vi "selectROI.vi"() -> ()   [LabVIEW 2010]
uses:
  <vilib>/Utility/miscctls.llb/LVPoint32TypeDef.ctl
  <vilib>/measure/NI_MABase.lvlib
panel:
  out "bottom":i32
  out "right":i32
  out "top":i32
  out "Left":i32
  out "bottom":i16
  out "right":i16
  out "top":i16
  out "left":i16
  in  "signal type":T1(ring)
  in  "amplitude":dbl(slide)=10.0 scale=0.0..10.0
  in  "frequency":dbl(slide)=9.923664122137405 scale=0.0..100.0
  in  "stop":bool
  out "Waveform Graph":waveform(dbl)(graph)={"t0"=timestamp(22.0 s since 1904-01-01), "dt"=0.001, "Y"=array[1000 elements]}
  # "plot bounds"
  # "ROI bounds"
  # "Define the graph rectangle by selecting an area with mouse"
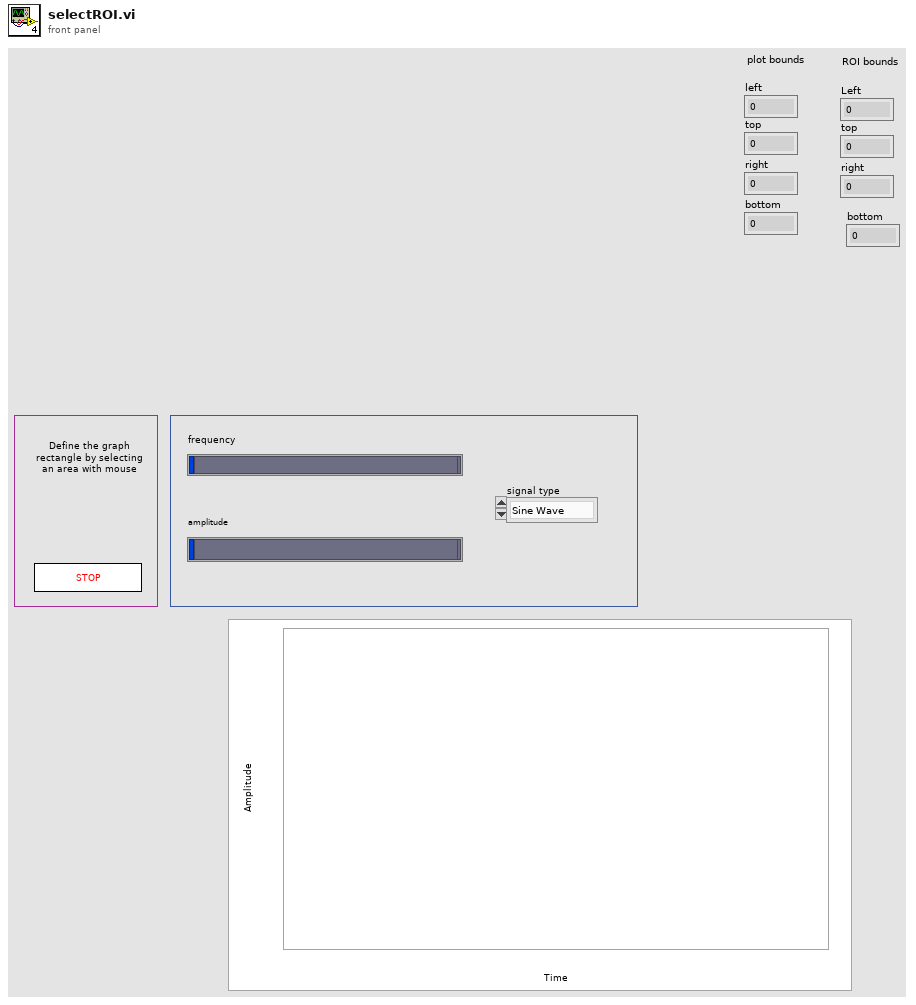
[diagram p1: front panel]
types:
  T1 = enum16{"Sine Wave", "Triangle Wave", "Square Wave", "Sawtooth Wave"}
  T2 = typedef "LVPoint32TypeDef.ctl" = cluster{"Horizontal":i32, "Vertical":i32}
  T3 = typedef "LVRectTypeDef.ctl" = cluster{"left":i16, "top":i16, "right":i16, "bottom":i16}
  T4 = cluster{"Width":i16, "Style":enum32{"Solid", "Dash", "Dot", "DashDot", "DashDotDot"}}
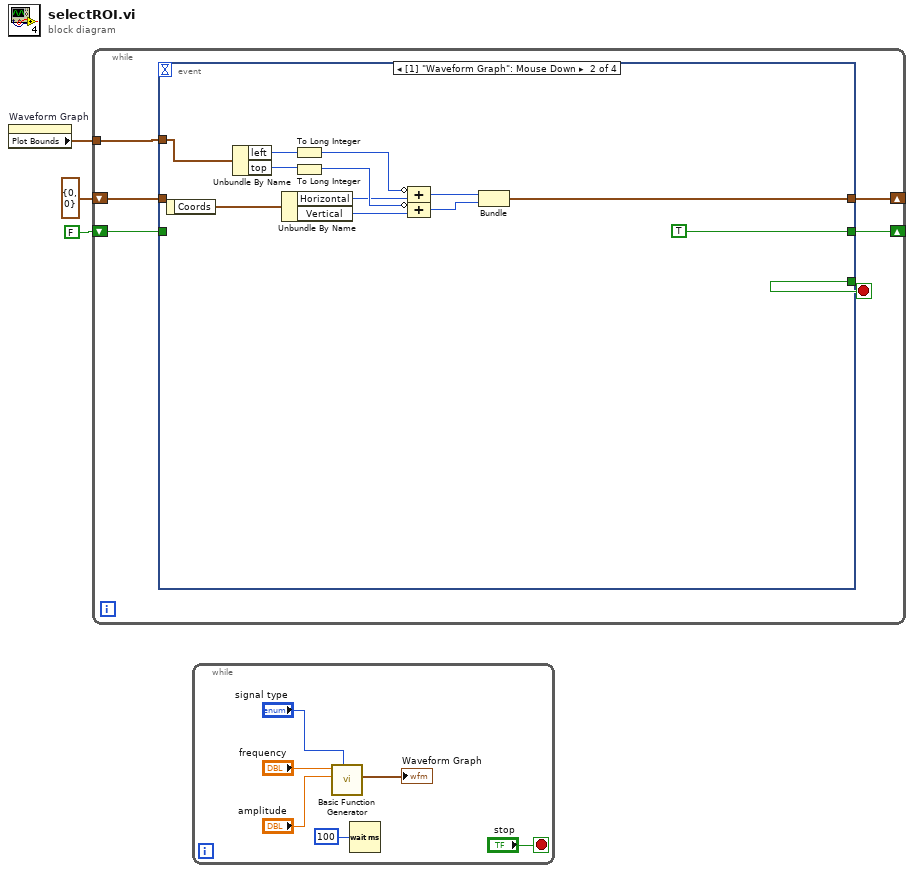
[diagram p0: block diagram]
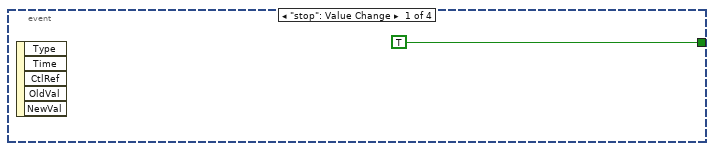
[diagram p2: hidden frame]
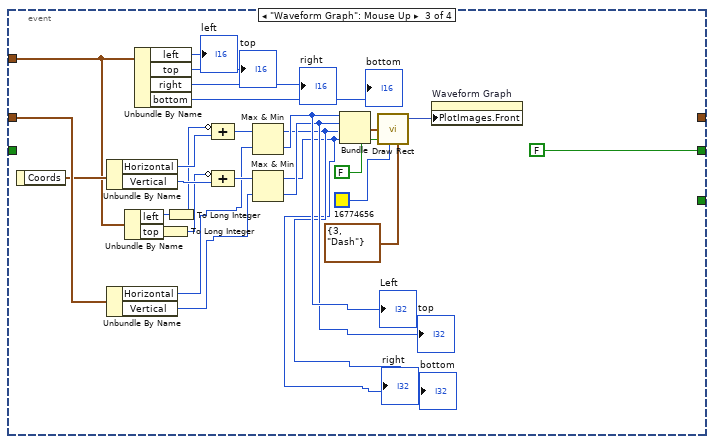
[diagram p3: hidden frame]
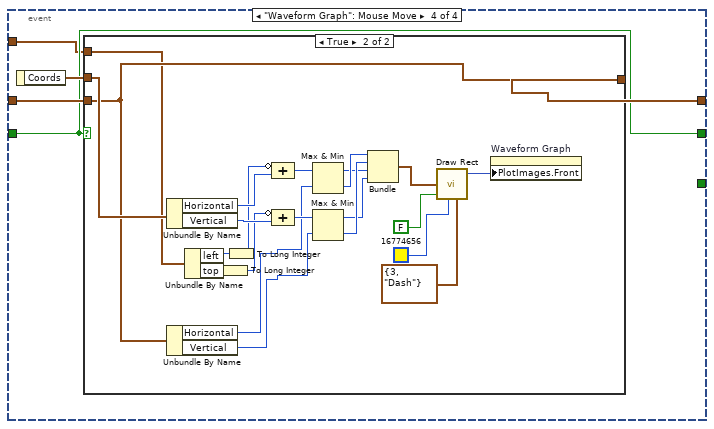
[diagram p4: hidden frame]
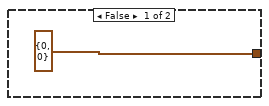
[diagram p5: hidden frame]
diagram:
  n1 = property on="Waveform Graph" class="WFGraph (strict)"() -> ("Plot Bounds"=w1:T3)  [unwired: 2 in, 2 out]
  n2 = while {
    shift-right: [w8] -> _
    shift-left: T2 {"Horizontal"=0, "Vertical"=0} ("Coords") -> [w5]
    shift-right: [w6] -> _
    shift-left: FALSE -> [w7]
    tunnel: w1 -> [w4]
    stop <- w9 stop-if-true
    n3 = event shown="[1] \"Waveform Graph\": Mouse Down" {
      selector: _ -> [_ _ _ _]
      dyn-events: _ -> [_ _ _ _]
      timeout: _ -> [_ _ _ _]
      tunnel: [TRUE _ _ _] -> w9
      tunnel: [_ w11 _ w52] -> w8
      tunnel: w5 -> [_ _ w38 w54]
      tunnel: w7 -> [_ _ _ w51]
      tunnel: [_ TRUE FALSE w51] -> w6
      tunnel: w4 -> [_ w16 w33 w50]
      event "stop": Value Change {
        n4 = event-data() -> ()  [unwired: 1 in, 5 out]
      }
      event "Waveform Graph": Mouse Down {
        n5 = event-data() -> ("Coords"=w21:T2)  [unwired: 1 in]
        n6 = Unbundle By Name(w16) -> ("left"=w20:i16, "top"=w18:i16)
        n7 = Unbundle By Name(w21) -> ("Horizontal"=w14:i32, "Vertical"=w15:i32)
        n8 = To Long Integer(number=w20) -> (32bit integer=w19:i32)
        n9 = To Long Integer(number=w18) -> (32bit integer=w17:i32)
        n10 = Compound Arithmetic op=ADD(invert w19, w14) -> (w13:i32)
        n11 = Compound Arithmetic op=ADD(invert w17, w15) -> (w12:i32)
        n12 = Bundle(w13, w12) -> (w11:cluster{i32, i32})  [unwired: 1 in]
      }
      event "Waveform Graph": Mouse Up {
        n13 = event-data() -> ("Coords"=w37:T2)  [unwired: 1 in]
        n14 = Unbundle By Name(w37) -> ("Horizontal"=w44:i32, "Vertical"=w42:i32)
        n15 = Unbundle By Name(w38) -> ("Horizontal"=w35:i32, "Vertical"=w34:i32)
        n16 = Unbundle By Name(w33) -> ("left"=w27:i16, "top"=w40:i16)
        n17 = Unbundle By Name(w33) -> ("left"=→"left":i16, "top"=→"top":i16, "right"=→"right":i16, "bottom"=→"bottom":i16)
        n18 = To Long Integer(number=w40) -> (32bit integer=w28:i32)
        n19 = To Long Integer(number=w27) -> (32bit integer=w36:i32)
        n20 = Compound Arithmetic op=ADD(invert w36, w44) -> (w43:i32)
        n21 = Compound Arithmetic op=ADD(invert w28, w42) -> (w41:i32)
        n22 = Max & Min(x=w43, y=w35) -> (max(x,y)=w24:i32, min(x,y)=w26:i32)
        "Left" <- w26
        "right" <- w24
        n23 = Max & Min(x=w41, y=w34) -> (max(x,y)=w23:i32, min(x,y)=w25:i32)
        "top" <- w25
        "bottom" <- w23
        n24 = Bundle(w26, w25, w24, w23) -> (w39:cluster{i32, i32, i32, i32})  [unwired: 1 out]
        n25 = call <vilib>:"Draw Rect.vi"("rect"=w39, "fill?(F)"=FALSE, "color(black)"=u32 16774656, "pen"=T4 {"Width"=3, "Style"=enum."Dash"}) -> ("new picture"=w47:picture)  [unwired: 5 in]
        n26 = property on="Waveform Graph" class="WFGraph (strict)"("PlotImages.Front"=w47) -> ()  [unwired: 2 in, 2 out]
      }
      event "Waveform Graph": Mouse Move {
        n27 = event-data() -> ("Coords"=w53:T2)  [unwired: 1 in]
        n28 = case shown="True" w51 {
          tunnel: w54 -> [_ w59]
          tunnel: w53 -> [_ w60]
          tunnel: [T2 {"Horizontal"=0, "Vertical"=0} ("Coords") w59] -> w52
          tunnel: w50 -> [_ w58]
          frame False {
          }
          frame True {
            n29 = Unbundle By Name(w60) -> ("Horizontal"=w69:i32, "Vertical"=w66:i32)
            n30 = Unbundle By Name(w59) -> ("Horizontal"=w57:i32, "Vertical"=w56:i32)
            n31 = Unbundle By Name(w58) -> ("left"=w67:i16, "top"=w64:i16)
            n32 = To Long Integer(number=w64) -> (32bit integer=w62:i32)
            n33 = To Long Integer(number=w67) -> (32bit integer=w63:i32)
            n34 = Compound Arithmetic op=ADD(invert w63, w69) -> (w68:i32)
            n35 = Compound Arithmetic op=ADD(invert w62, w66) -> (w65:i32)
            n36 = Max & Min(x=w68, y=w57) -> (max(x,y)=w70:i32, min(x,y)=w73:i32)
            n37 = Max & Min(x=w65, y=w56) -> (max(x,y)=w71:i32, min(x,y)=w72:i32)
            n38 = Bundle(w73, w72, w70, w71) -> (w61:cluster{i32, i32, i32, i32})  [unwired: 1 out]
            n39 = call <vilib>:"Draw Rect.vi"("rect"=w61, "fill?(F)"=FALSE, "color(black)"=u32 16774656, "pen"=T4 {"Width"=3, "Style"=enum."Dash"}) -> ("new picture"=w75:picture)  [unwired: 5 in]
            n40 = property on="Waveform Graph" class="WFGraph (strict)"("PlotImages.Front"=w75) -> ()  [unwired: 2 in, 2 out]
          }
        }
      }
    }
  }
  n41 = while {
    stop <- "stop" stop-if-true
    n42 = call <vilib>:"Basic Function Generator.vi"("signal type"="signal type", "amplitude"="amplitude", "frequency"="frequency") -> ("signal out"=→"Waveform Graph":waveform(dbl))  [unwired: 6 in, 2 out]
    n43 = Wait (ms)(milliseconds to wait=u32 100) -> ()  [unwired: 1 out]
  }
